vi "NML Spectrum Conversion.vi"(3 "Filter Type":T1(ring), 4 "DELTA TIME µSec":i32=25, 5 "WAVEFORM DATA":dbl[](array[numeric]) format="%.2f") -> (0 "FREQUENCY \nRESOLUTION":dbl format="%.4f", 1 "SPECTRUM DATA":dbl[](array[numeric]) format="%.8f", 2 "SPECTRUM":cluster{ext, dbl, dbl[]}(graph))   [LabVIEW 2020]
uses:
  <vilib>/Analysis/4window.llb/Hanning Window (DBL).vi
  <vilib>/Analysis/4window.llb/Hamming Window (DBL).vi
  <vilib>/Analysis/4window.llb/Kaiser-Bessel Window (DBL).vi
  <vilib>/Analysis/4window.llb/Flat Top Window (DBL).vi
  <vilib>/Analysis/4window.llb/Triangle Window (DBL).vi
  <vilib>/Analysis/4window.llb/General Cosine Window (DBL).vi
  <vilib>/Analysis/4window.llb/Cosine Tapered Window (DBL).vi
  <vilib>/Analysis/4window.llb/Blackman Window (DBL).vi
  <vilib>/Analysis/4window.llb/Exact Blackman Window (DBL).vi
  <vilib>/Analysis/4window.llb/Blackman-Harris Window (DBL).vi
  <vilib>/Analysis/2dsp.llb/Power Spectrum (DBL).vi
  <vilib>/Analysis/4window.llb/AllCosWindow (DBL).vi
  <vilib>/Analysis/NI_AALPro.lvlib
panel:
  # "dB"
  # "Hz"
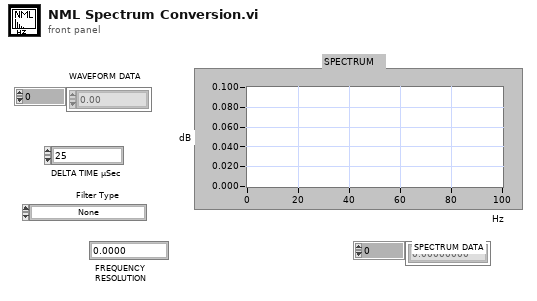
[diagram p1: front panel]
types:
  T1 = enum16{"None", "Hanning", "Hamming", "Kaiser-Bessel", "Flat Top", "Triangle", "Genral Cosine", "Cosine Tapered", "Blackman", "Exact Blackman", "Blackman-Harris"}
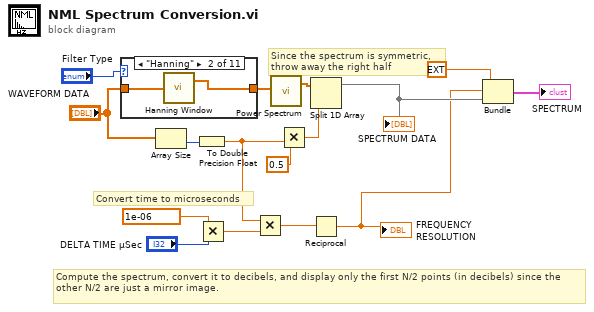
[diagram p0: block diagram]
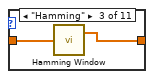
[diagram p3: hidden frame]
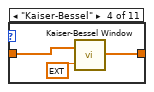
[diagram p4: hidden frame]
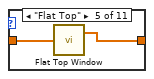
[diagram p5: hidden frame]
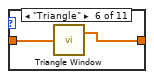
[diagram p6: hidden frame]
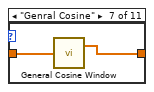
[diagram p7: hidden frame]
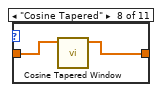
[diagram p8: hidden frame]
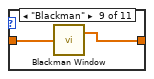
[diagram p9: hidden frame]
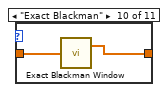
[diagram p10: hidden frame]
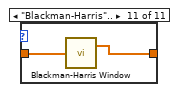
[diagram p11: hidden frame]
diagram:
  # "Compute the spectrum, convert it to decibels, and display only the first N/2 points (in decibels) since the other N/2 are just a mirror image."
  # "Since the spectrum is symmetric,\nthrow away the right half"
  # "Convert time to microseconds"
  n1 = case shown="\"Hanning\"" "Filter Type" {
    tunnel: [w17 w18 w20 w24 w25 w27 w29 w31 w33 w35 w37] -> w7
    tunnel: "WAVEFORM DATA" -> [w17 w19 w21 w23 w26 w28 w30 w32 w34 w36 w38]
    frame .."None" {
    }
    frame "Hanning" {
      n2 = call-poly <vilib>:"Hanning Window.vi"("X"=w19) -> ("Windowed X"=w18:dbl[])  [unwired: 1 out]
    }
    frame "Hamming" {
      n3 = call-poly <vilib>:"Hamming Window.vi"("X"=w21) -> ("Windowed X"=w20:dbl[])  [unwired: 1 out]
    }
    frame "Kaiser-Bessel" {
      n4 = call-poly <vilib>:"Kaiser-Bessel Window.vi"("beta"=ext 0.5, "X"=w23) -> ("Windowed X"=w24:dbl[])  [unwired: 1 out]
    }
    frame "Flat Top" {
      n5 = call-poly <vilib>:"Flat Top Window.vi"("X"=w26) -> ("Windowed X"=w25:dbl[])  [unwired: 1 out]
    }
    frame "Triangle" {
      n6 = call-poly <vilib>:"Triangle Window.vi"("X"=w28) -> ("Windowed X"=w27:dbl[])  [unwired: 1 out]
    }
    frame "Genral Cosine" {
      n7 = call-poly <vilib>:"General Cosine Window.vi"("Cosine Coefficients"=w30) -> ("Windowed X"=w29:dbl[])  [unwired: 1 in, 1 out]
    }
    frame "Cosine Tapered" {
      n8 = call-poly <vilib>:"Cosine Tapered Window.vi"("X"=w32) -> ("Windowed X"=w31:dbl[])  [unwired: 9 in, 1 out]
    }
    frame "Blackman" {
      n9 = call-poly <vilib>:"Blackman Window.vi"("X"=w34) -> ("Windowed X"=w33:dbl[])  [unwired: 1 out]
    }
    frame "Exact Blackman" {
      n10 = call-poly <vilib>:"Exact Blackman Window.vi"("X"=w36) -> ("Windowed X"=w35:dbl[])  [unwired: 1 out]
    }
    frame "Blackman-Harris".. {
      n11 = call-poly <vilib>:"Blackman-Harris Window.vi"("X"=w38) -> ("Windowed X"=w37:dbl[])  [unwired: 1 out]
    }
  }
  n12 = Array Size(array="WAVEFORM DATA") -> (size(s)=w14:i32)
  n13 = To Double Precision Float(number=w14) -> (double precision float=w5:dbl)
  n14 = Multiply(x=1e-06, y="DELTA TIME µSec") -> (x*y=w11:dbl)
  n15 = Multiply(x=w5, y=w11) -> (x*y=w15:dbl)
  n16 = call-poly <vilib>:"Power Spectrum.vi"("X"=w7) -> ("Power Spectrum"=w12:dbl[])  [unwired: 1 out]
  n17 = Multiply(x=w5, y=0.5) -> (x*y=w13:dbl)
  n18 = Split 1D Array(array=w12, index=w13) -> (first subarray=w3:dbl[])  [unwired: 1 out]
  "SPECTRUM DATA" <- w3
  n19 = Reciprocal(x=w15) -> (1/x=w1:dbl)
  "FREQUENCY \nRESOLUTION" <- w1
  n20 = Bundle(ext 0.0, w1, w3) -> (→"SPECTRUM":cluster{ext, dbl, dbl[]})  [unwired: 1 in]
